vi "StepRead.vi"(5 "Data Read":string, 7 "Cluster in":T2) -> (8 "Results":T1)   [LabVIEW 2023]
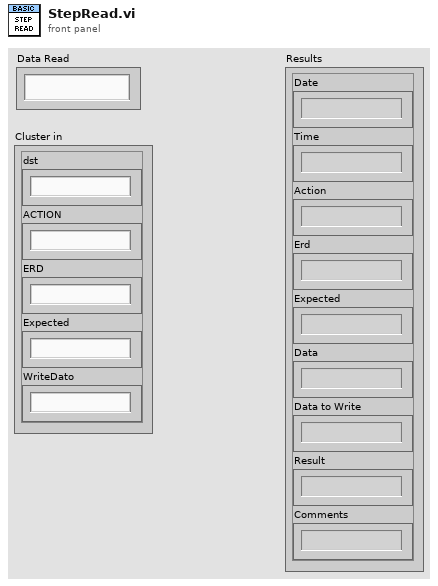
[diagram p1: front panel]
types:
  T1 = cluster{"Date":string, "Time":string, "Action":string, "Erd":string, "Expected":string, "Data":string, "Data to Write":string, "Result":string, "Comments":string}
  T2 = cluster{"dst":string, "ACTION":string, "ERD":string, "Expected":string, "WriteDato":string}
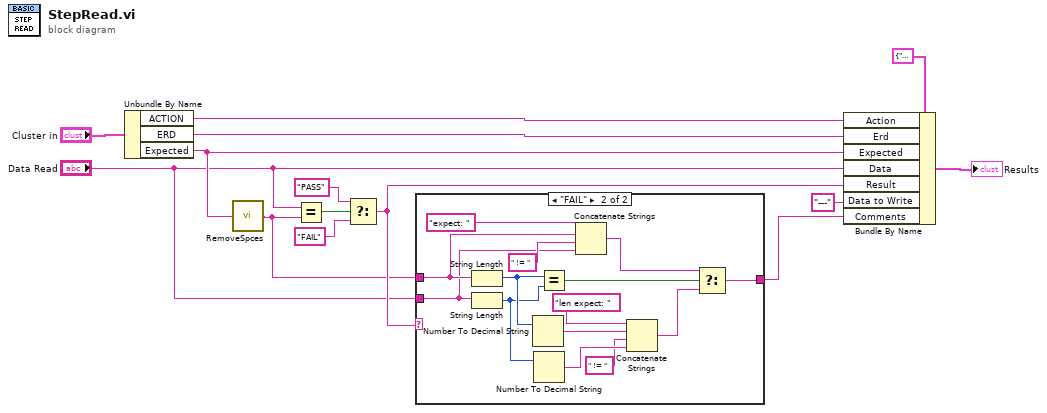
[diagram p0: block diagram]
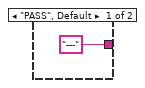
[diagram p2: hidden frame]
diagram:
  n1 = Unbundle By Name("Cluster in") -> ("ACTION"=w9:string, "ERD"=w8:string, "Expected"=w7:string)
  n2 = call "RemoveSpces.vi"("input string"=w7) -> ("result string"=w3:string)  [unwired: 14 in]
  n3 = Equal?(x="Data Read", y=w3) -> (x = y?=w13:bool)
  n4 = Select(t="PASS", s=w13, f="FAIL") -> (s? t:f=w5:string)
  n5 = case shown="\"FAIL\"" w5 {
    tunnel: ["---" ("Data to Write") w16] -> w2
    tunnel: "Data Read" -> [_ w24]
    tunnel: w3 -> [_ w26]
    frame "PASS", Default {
    }
    frame "FAIL" {
      n6 = String Length(string=w26) -> (length=w23:i32)
      n7 = String Length(string=w24) -> (length=w22:i32)
      n8 = Number To Decimal String(number=w23) -> (decimal integer string=w20:string)  [unwired: 1 in]
      n9 = Number To Decimal String(number=w22) -> (decimal integer string=w19:string)  [unwired: 1 in]
      n10 = Equal?(x=w23, y=w22) -> (x = y?=w29:bool)
      n11 = Concatenate Strings("expect: ", w26, " != ", w24) -> (w28:string)
      n12 = Concatenate Strings("len expect: " ("string"), w20, " != ", w19) -> (w17:string)
      n13 = Select(t=w28, s=w29, f=w17) -> (s? t:f=w16:string)
    }
  }
  n14 = Bundle By Name(cluster=T1 {"Date"="", "Time"="", "Action"="", "Erd"="", "Expected"="", "Data"="", "Data to Write"="", "Result"="", "Comments"=""}, "Action"=w9, "Erd"=w8, "Expected"=w7, "Data"="Data Read", "Result"=w5, "Data to Write"="---", "Comments"=w2) -> (→"Results":T1)
